vi "DataGrid for LabVIEW Documentation....vi"   [LabVIEW 2013]
panel:
  # "This VI simply opens the documentation page on github for the addon"
  # "NOTE:  No Support is provided directly for this add-on, since its a free product, but             you can use the community github page or the LabVIEW forums for help and questions"
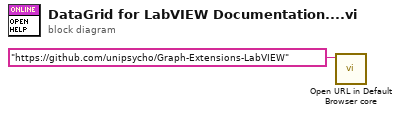
[diagram p0: block diagram]
diagram:
  n1 = call <vilib>:"Open URL in Default Browser core.vi"("url"="https://github.com/unipsycho/Graph-Extensions-LabVIEW") -> ()  [unwired: 5 in, 2 out]
